vi "Read Axis Position data.vi"(8 "error in (no error)":errorcluster, 11 "Fiber Auto Collimation state data in":refnum<class "Fiber Auto Collimation state data.lvclass">) -> (0 "error out":errorcluster, 2 "Current position":dbl[unit], 3 "Fiber Auto Collimation state data out":refnum<class "Fiber Auto Collimation state data.lvclass">)   [LabVIEW 2018, in "Fiber Auto Collimation state data.lvclass"]
doc: "This \"LIV test data\" is just a placeholder and example for how real test data might be stored. This accessor plus its data in the state data class private control probably need to be removed or replaced with something to hold test data for the actual station."
uses:
  Fiber Auto Collimation state data.lvclass
  Fiber Auto Collimation state data.lvclass/Fiber Auto Collimation state data.ctl
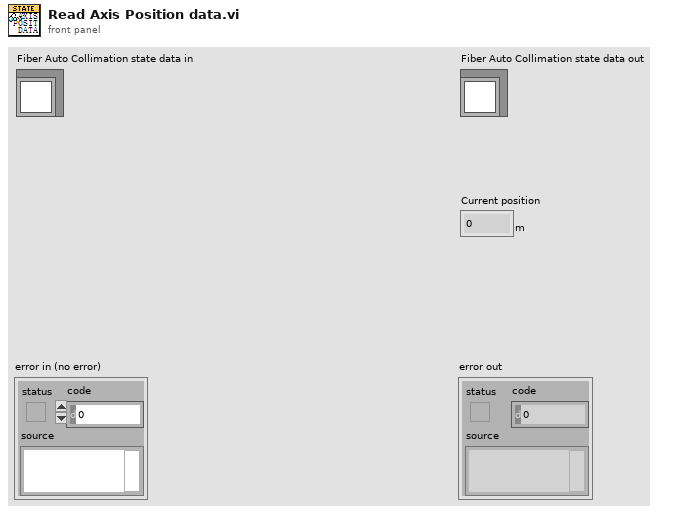
[diagram p1: front panel]
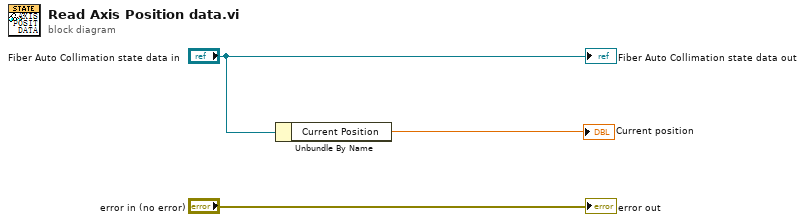
[diagram p0: block diagram]
diagram:
  n1 = Unbundle By Name("Fiber Auto Collimation state data in") -> ("Current Position"=→"Current position":dbl[unit])
  "error out" <- "error in (no error)"
  "Fiber Auto Collimation state data out" <- "Fiber Auto Collimation state data in"
